vi "Read connFlags.vi"(8 "error in (no error)":errorcluster, 11 "mqtt in":refnum<class "MQTT Client.lvclass">) -> (0 "error out":errorcluster, 2 "connFlags":T1, 3 "mqtt out":refnum<class "MQTT Client.lvclass">)   [LabVIEW 2020, in "MQTT Client.lvclass"]
uses:
  MQTT Client.lvclass
  mqttTypedef/mqttConnectionFlags.ctl
  MQTT Client.lvclass/MQTT Client.ctl
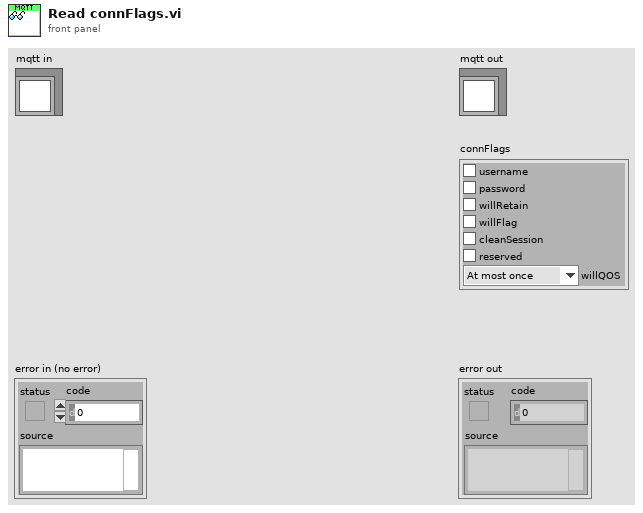
[diagram p1: front panel]
types:
  T1 = typedef "MQTT Client.lvclass/mqttConnectionFlags.ctl" = cluster{"user name":bool, "password":bool, "will retain":bool, "will flag":bool, "clean session":bool, "reserved":bool, "willQOS":enum8{"At most once", "At least once", "Exactly once", "Reserved"}}
  T2 = typedef "mqtt.lvclass/mqttConnectionFlags.ctl" = cluster{"user name":bool, "password":bool, "will retain":bool, "will flag":bool, "clean session":bool, "reserved":bool, "willQOS":enum8{"At most once", "At least once", "Exactly once", "Reserved"}}
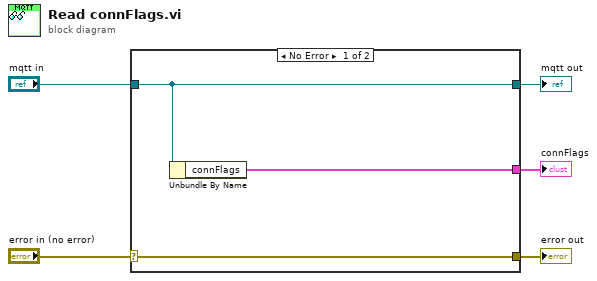
[diagram p0: block diagram]
diagram:
  n1 = case shown="No Error" "error in (no error)" {
    selector: "error in (no error)" -> [w8 w9]
    tunnel: [w8 w9] -> w4
    tunnel: [w7 w10] -> w2
    tunnel: "mqtt in" -> [w7 w10]
    tunnel: [w6 _] -> w1
    frame No Error {
      n2 = Unbundle By Name(w7) -> ("connFlags"=w6:T2)
    }
    frame Error {
    }
  }
  "error out" <- w4
  "mqtt out" <- w2
  "connFlags" <- w1
